vi "Advance past Number.vi"(7 "JSON":string, 9 "Offset (0)":i32, 11 "Parser State in":T2=enum."Number/Other") -> (1 "Offset past match":i32, 3 "Parser State":T2, 4 "JSON Value Type":T1, 6 "Value start out":i32)   [LabVIEW 2019, in "JSONtext.lvlib"]
uses:
  JSONtext.lvlib
  Parsing State.ctl
  JSON Value Type.ctl
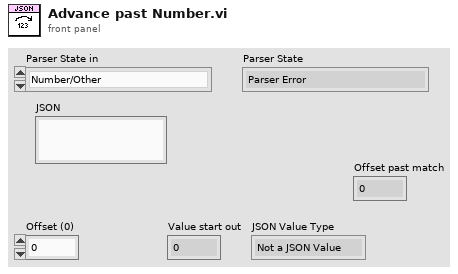
[diagram p1: front panel]
types:
  T1 = typedef "JSONtext.lvlib/JSON Value Type.ctl" = enum16{"Not a JSON Value", "JSON Object", "JSON Array", "String", "Number", "true", "false", "null"}
  T2 = typedef "JSONtext.lvlib/Parsing State.ctl" = enum16{"Parser Error", "Object", "Array", "String", "Number/Other", "Leading Whitespace", "Object end", "Array end", "Value end"}
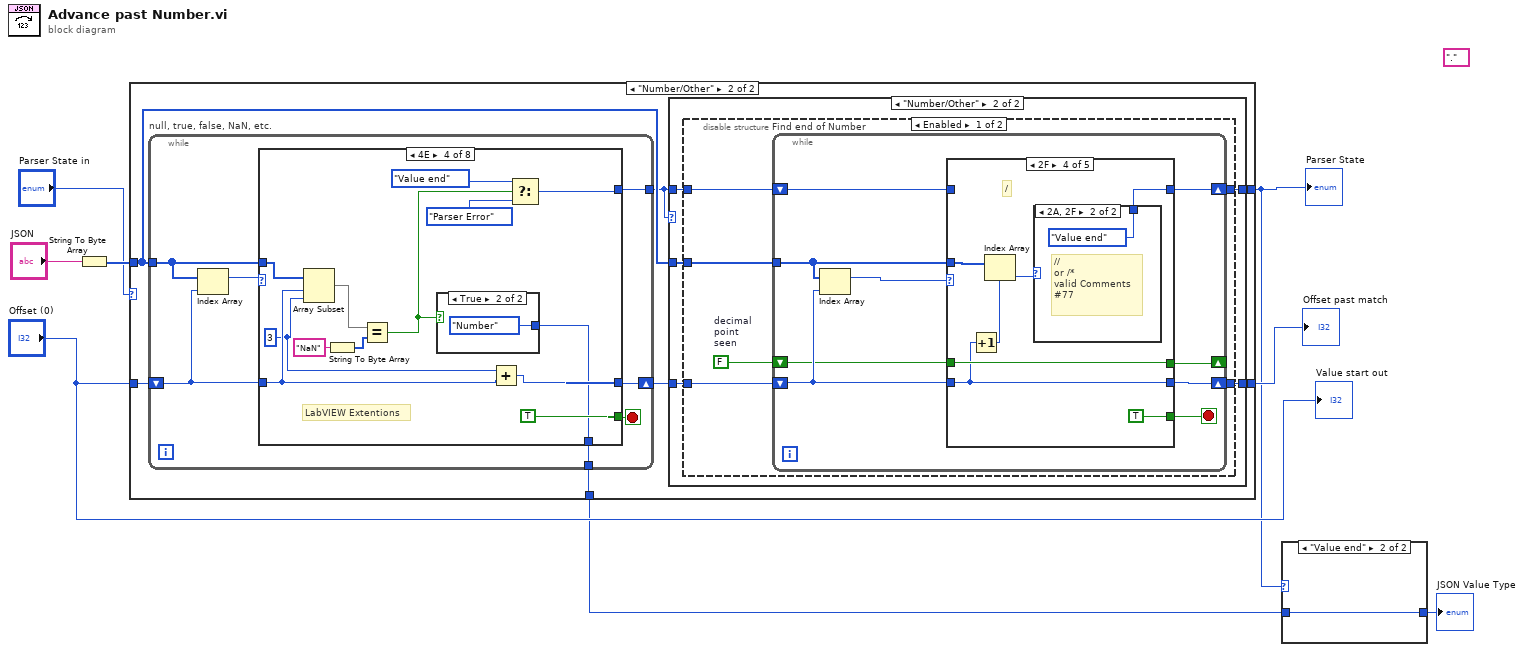
[diagram p0: block diagram]
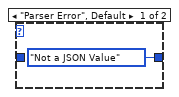
[diagram p2: hidden frame]
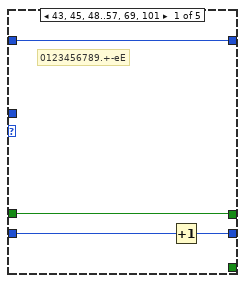
[diagram p5: hidden frame]
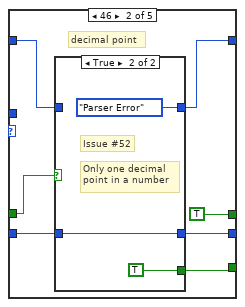
[diagram p6: hidden frame]
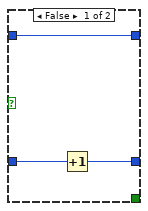
[diagram p7: hidden frame]
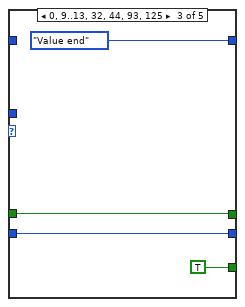
[diagram p8: hidden frame]
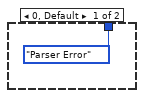
[diagram p9: hidden frame]
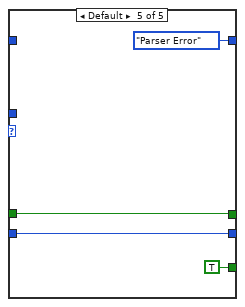
[diagram p10: hidden frame]
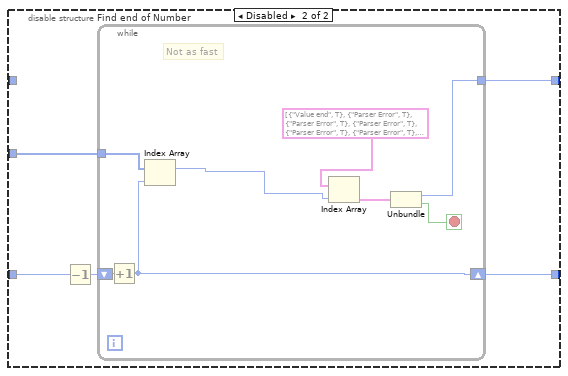
[diagram p11: hidden frame]
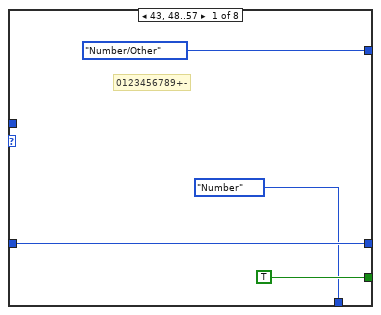
[diagram p12: hidden frame]
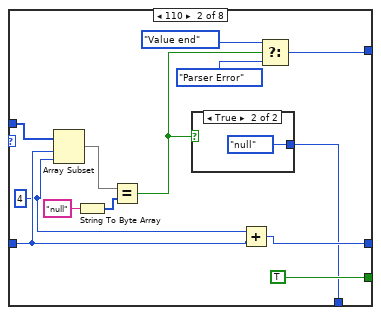
[diagram p13: hidden frame]
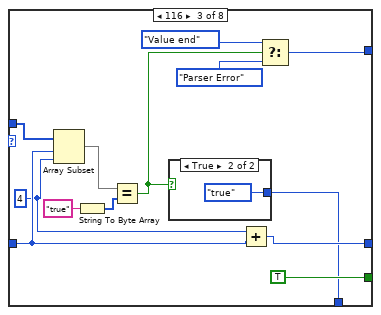
[diagram p15: hidden frame]
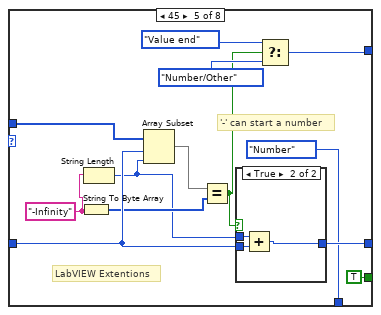
[diagram p18: hidden frame]
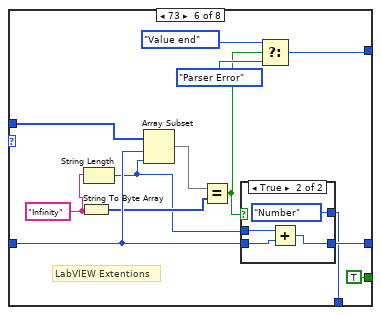
[diagram p20: hidden frame]
diagram:
  (unwired) "."
  n1 = String To Byte Array(string="JSON") -> (unsigned byte array=w5:u8[])
  n2 = case shown="\"Number/Other\"" "Parser State in" {
    tunnel: [_ w16] -> w3
    tunnel: [w9 w15] -> w8
    tunnel: w5 -> [_ w13]
    tunnel: "Offset (0)" -> [w9 w11]
    tunnel: [_ w10] -> w2
    frame "Parser Error", Default {
    }
    frame "Number/Other" {
      n3 = while "null, true, false, NaN, etc." {
        tunnel: w13 -> [w91]
        shift-right: [w87] -> w14
        shift-left: w11 -> [w88]
        tunnel: [w90] -> w12
        tunnel: [w86] -> w10
        stop <- w89 stop-if-true
        n4 = Index Array(array=w91, index=w88) -> (element=w92:u8)
        n5 = case shown="4E" w92 {
          tunnel: w91 -> [_ w108 w122 w136 w151 w168 w185 _]
          tunnel: [Parsing_State."Number/Other" w105 w119 w133 w149 w166 w182 Parsing_State."Parser Error"] -> w90
          tunnel: [TRUE TRUE TRUE TRUE TRUE TRUE TRUE TRUE] -> w89
          tunnel: w88 -> [w94 w101 w115 w129 w145 w162 w178 w191]
          tunnel: [w94 w99 w113 w127 w144 w161 w176 w191] -> w87
          tunnel: [JSON_Value_Type."Number" w97 w111 w125 JSON_Value_Type."Number" w156 w174 JSON_Value_Type."Not a JSON Value"] -> w86
          frame 43, 48..57 {
            # "0123456789+-"
          }
          frame 110 {
            w100 = 4 ("length")
            n6 = Array Subset(array=w108, index=w101, length=w100) -> (w106:u8[])
            n7 = String To Byte Array(string="null") -> (unsigned byte array=w107:u8[])
            n8 = Equal?(x=w106, y=w107) -> (x = y?=w98:bool)
            n9 = case shown="True" w98 {
              tunnel: [_ JSON_Value_Type."null"] -> w97
              frame False {
              }
              frame True {
              }
            }
            n10 = Add(x=w100, y=w101) -> (x+y=w99:i32)
            n11 = Select(t=Parsing_State."Value end", s=w98, f=Parsing_State."Parser Error") -> (s? t:f=w105:T2)
          }
          frame 116 {
            w114 = 4 ("length")
            n12 = Array Subset(array=w122, index=w115, length=w114) -> (w120:u8[])
            n13 = String To Byte Array(string="true") -> (unsigned byte array=w121:u8[])
            n14 = Equal?(x=w120, y=w121) -> (x = y?=w112:bool)
            n15 = case shown="True" w112 {
              tunnel: [_ JSON_Value_Type."true"] -> w111
              frame False {
              }
              frame True {
              }
            }
            n16 = Add(x=w114, y=w115) -> (x+y=w113:i32)
            n17 = Select(t=Parsing_State."Value end", s=w112, f=Parsing_State."Parser Error") -> (s? t:f=w119:T2)
          }
          frame 78 {
            w128 = 3 ("length")
            # "LabVIEW Extentions"
            n18 = Array Subset(array=w136, index=w129, length=w128) -> (w134:u8[])
            n19 = String To Byte Array(string="NaN") -> (unsigned byte array=w135:u8[])
            n20 = Equal?(x=w134, y=w135) -> (x = y?=w126:bool)
            n21 = case shown="True" w126 {
              tunnel: [_ JSON_Value_Type."Number"] -> w125
              frame False {
              }
              frame True {
              }
            }
            n22 = Add(x=w128, y=w129) -> (x+y=w127:i32)
            n23 = Select(t=Parsing_State."Value end", s=w126, f=Parsing_State."Parser Error") -> (s? t:f=w133:T2)
          }
          frame 45 {
            w142 = "-Infinity"
            # "'-' can start a number"
            # "LabVIEW Extentions"
            n24 = String To Byte Array(string=w142) -> (unsigned byte array=w143:u8[])
            n25 = String Length(string=w142) -> (length=w141:i32)
            n26 = Array Subset(array=w151, index=w145, length=w141) -> (w150:u8[])
            n27 = Equal?(x=w150, y=w143) -> (x = y?=w140:bool)
            n28 = case shown="True" w140 {
              tunnel: w145 -> [w152 w155]
              tunnel: [w152 w154] -> w144
              tunnel: w141 -> [_ w153]
              frame False {
              }
              frame True {
                n29 = Add(x=w153, y=w155) -> (x+y=w154:i32)
              }
            }
            n30 = Select(t=Parsing_State."Value end", s=w140, f=Parsing_State."Number/Other") -> (s? t:f=w149:T2)
          }
          frame 73 {
            w159 = "Infinity"
            # "LabVIEW Extentions"
            n31 = String To Byte Array(string=w159) -> (unsigned byte array=w160:u8[])
            n32 = String Length(string=w159) -> (length=w158:i32)
            n33 = Array Subset(array=w168, index=w162, length=w158) -> (w167:u8[])
            n34 = Equal?(x=w167, y=w160) -> (x = y?=w157:bool)
            n35 = case shown="True" w157 {
              tunnel: w162 -> [w169 w173]
              tunnel: [w169 w172] -> w161
              tunnel: w158 -> [_ w171]
              tunnel: [_ JSON_Value_Type."Number"] -> w156
              frame False {
              }
              frame True {
                n36 = Add(x=w171, y=w173) -> (x+y=w172:i32)
              }
            }
            n37 = Select(t=Parsing_State."Value end", s=w157, f=Parsing_State."Parser Error") -> (s? t:f=w166:T2)
          }
          frame 102 {
            w177 = 5 ("length")
            n38 = Array Subset(array=w185, index=w178, length=w177) -> (w183:u8[])
            n39 = String To Byte Array(string="false") -> (unsigned byte array=w184:u8[])
            n40 = Equal?(x=w183, y=w184) -> (x = y?=w175:bool)
            n41 = case shown="True" w175 {
              tunnel: [_ JSON_Value_Type."false"] -> w174
              frame False {
              }
              frame True {
              }
            }
            n42 = Add(x=w177, y=w178) -> (x+y=w176:i32)
            n43 = Select(t=Parsing_State."Value end", s=w175, f=Parsing_State."Parser Error") -> (s? t:f=w182:T2)
          }
          frame Default {
          }
        }
      }
      n44 = case shown="\"Number/Other\"" w12 {
        tunnel: [w17 w23] -> w16
        tunnel: [w18 w22] -> w15
        tunnel: w14 -> [w18 w19]
        tunnel: w12 -> [w17 w21]
        tunnel: w13 -> [_ w20]
        frame "Parser Error", Default {
        }
        frame "Number/Other" {
          n45 = disable-structure shown="Enabled" {
            disable-tunnel: [w29 w77] -> w23
            disable-tunnel: [w28 w76] -> w22
            disable-tunnel: w21 -> [w27 _]
            disable-tunnel: w20 -> [w26 w75]
            disable-tunnel: w19 -> [w25 w74]
            frame Enabled {
              w24 = FALSE  # decimal point seen
              n46 = while "Find end of Number" {
                tunnel: w26 -> [w38]
                shift-right: [w34] -> w28
                shift-left: w25 -> [w32]
                shift-right: [w36] -> w29
                shift-left: w27 -> [w37]
                shift-right: [w31] -> _
                shift-left: w24 -> [w30]
                stop <- w35 stop-if-true
                n47 = Index Array(array=w38, index=w32) -> (element=w33:u8)
                n48 = case shown="2F" w33 {
                  tunnel: w38 -> [_ _ _ w62 _]
                  tunnel: w37 -> [w42 w45 _ _ _]
                  tunnel: [w42 w44 Parsing_State."Value end" w60 Parsing_State."Parser Error"] -> w36
                  tunnel: [_ w43 TRUE TRUE TRUE] -> w35
                  tunnel: w32 -> [w41 w49 w57 w64 w72]
                  tunnel: [w40 w48 w57 w64 w72] -> w34
                  tunnel: [w39 TRUE w56 w65 w69] -> w31
                  tunnel: w30 -> [w39 w46 w56 w65 w69]
                  frame 43, 45, 48..57, 69, 101 {
                    # "0123456789.+-eE"
                    n49 = Increment(x=w41) -> (x+1=w40:i32)
                  }
                  frame 46 {
                    # "decimal point"
                    n50 = case shown="True" w46 {
                      tunnel: w49 -> [w52 w54]
                      tunnel: [w51 w54] -> w48
                      tunnel: [w50 Parsing_State."Parser Error"] -> w44
                      tunnel: w45 -> [w50 _]
                      tunnel: [_ TRUE] -> w43
                      frame False {
                        n51 = Increment(x=w52) -> (x+1=w51:i32)
                      }
                      frame True {
                        # "Only one decimal\npoint in a number"
                        # "Issue #52"
                      }
                    }
                  }
                  frame 0, 9..13, 32, 44, 93, 125 {
                  }
                  frame 47 {
                    # "/"
                    n52 = Increment(x=w64) -> (x+1=w63:i32)
                    n53 = Index Array(array=w62, index=w63) -> (element=w61:u8)
                    n54 = case shown="2A, 2F" w61 {
                      tunnel: [Parsing_State."Parser Error" Parsing_State."Value end"] -> w60
                      frame 0, Default {
                      }
                      frame 42, 47 {
                        # "//\nor /*\nvalid Comments\n#77"
                      }
                    }
                  }
                  frame Default {
                  }
                }
              }
            }
            frame Disabled {
              n55 = Decrement(x=w74) -> (x-1=w73:i32)
              n56 = while "Find end of Number" {
                tunnel: w75 -> [w85]
                shift-right: [w78] -> w76
                shift-left: w73 -> [w84]
                tunnel: [w79] -> w77
                stop <- w80 stop-if-true
                # "Not as fast"
                n57 = Increment(x=w84) -> (x+1=w78:i32)
                n58 = Index Array(array=w85, index=w78) -> (element=w81:u8)
                n59 = Index Array(array=cluster{T2, bool}[] [{enum."Value end", TRUE}, {enum."Parser Error", TRUE}, {enum."Parser Error", TRUE}, {enum."Parser Error", TRUE}, {enum."Parser Error", TRUE}, {enum."Parser Error", TRUE}, {enum."Parser Error", TRUE}, {enum."Parser Error", TRUE}, {enum."Parser Error", TRUE}, {enum."Value end", TRUE}, {enum."Value end", TRUE}, {enum."Value end", TRUE}, {enum."Value end", TRUE}, {enum."Value end", TRUE}, {enum."Parser Error", TRUE}, {enum."Parser Error", TRUE}, {enum."Parser Error", TRUE}, {enum."Parser Error", TRUE}, {enum."Parser Error", TRUE}, {enum."Parser Error", TRUE}, {enum."Parser Error", TRUE}, {enum."Parser Error", TRUE}, {enum."Parser Error", TRUE}, {enum."Parser Error", TRUE}, {enum."Parser Error", TRUE}, {enum."Parser Error", TRUE}, {enum."Parser Error", TRUE}, {enum."Parser Error", TRUE}, {enum."Parser Error", TRUE}, {enum."Parser Error", TRUE}, {enum."Parser Error", TRUE}, {enum."Parser Error", TRUE}, {enum."Value end", TRUE}, {enum."Parser Error", TRUE}, {enum."Parser Error", TRUE}, {enum."Parser Error", TRUE}, {enum."Parser Error", TRUE}, {enum."Parser Error", TRUE}, {enum."Parser Error", TRUE}, {enum."Parser Error", TRUE}, {enum."Parser Error", TRUE}, {enum."Parser Error", TRUE}, {enum."Parser Error", TRUE}, {enum."Number/Other", FALSE}, {enum."Value end", TRUE}, {enum."Number/Other", FALSE}, {enum."Number/Other", FALSE}, {enum."Parser Error", TRUE}, {enum."Number/Other", FALSE}, {enum."Number/Other", FALSE}, {enum."Number/Other", FALSE}, {enum."Number/Other", FALSE}, {enum."Number/Other", FALSE}, {enum."Number/Other", FALSE}, {enum."Number/Other", FALSE}, {enum."Number/Other", FALSE}, {enum."Number/Other", FALSE}, {enum."Number/Other", FALSE}, {enum."Parser Error", TRUE}, {enum."Parser Error", TRUE}, {enum."Parser Error", TRUE}, {enum."Parser Error", TRUE}, {enum."Parser Error", TRUE}, {enum."Parser Error", TRUE}, {enum."Parser Error", TRUE}, {enum."Parser Error", TRUE}, {enum."Parser Error", TRUE}, {enum."Parser Error", TRUE}, {enum."Parser Error", TRUE}, {enum."Number/Other", FALSE}, {enum."Parser Error", TRUE}, {enum."Parser Error", TRUE}, {enum."Parser Error", TRUE}, {enum."Parser Error", TRUE}, {enum."Parser Error", TRUE}, {enum."Parser Error", TRUE}, {enum."Parser Error", TRUE}, {enum."Parser Error", TRUE}, {enum."Parser Error", TRUE}, {enum."Parser Error", TRUE}, {enum."Parser Error", TRUE}, {enum."Parser Error", TRUE}, {enum."Parser Error", TRUE}, {enum."Parser Error", TRUE}, {enum."Parser Error", TRUE}, {enum."Parser Error", TRUE}, {enum."Parser Error", TRUE}, {enum."Parser Error", TRUE}, {enum."Parser Error", TRUE}, {enum."Parser Error", TRUE}, {enum."Parser Error", TRUE}, {enum."Parser Error", TRUE}, {enum."Parser Error", TRUE}, {enum."Value end", TRUE}, {enum."Parser Error", TRUE}, {enum."Parser Error", TRUE}, {enum."Parser Error", TRUE}, {enum."Parser Error", TRUE}, {enum."Parser Error", TRUE}, {enum."Parser Error", TRUE}, {enum."Parser Error", TRUE}, {enum."Number/Other", FALSE}, {enum."Parser Error", TRUE}, {enum."Parser Error", TRUE}, {enum."Parser Error", TRUE}, {enum."Parser Error", TRUE}, {enum."Parser Error", TRUE}, {enum."Parser Error", TRUE}, {enum."Parser Error", TRUE}, {enum."Parser Error", TRUE}, {enum."Parser Error", TRUE}, {enum."Parser Error", TRUE}, {enum."Parser Error", TRUE}, {enum."Parser Error", TRUE}, {enum."Parser Error", TRUE}, {enum."Parser Error", TRUE}, {enum."Parser Error", TRUE}, {enum."Parser Error", TRUE}, {enum."Parser Error", TRUE}, {enum."Parser Error", TRUE}, {enum."Parser Error", TRUE}, {enum."Parser Error", TRUE}, {enum."Parser Error", TRUE}, {enum."Parser Error", TRUE}, {enum."Parser Error", TRUE}, {enum."Value end", TRUE}] ("Array"), index=w81) -> (element=w82:cluster{T2, bool})
                n60 = Unbundle(w82) -> (w79:T2, w80:bool)
              }
            }
          }
        }
      }
    }
  }
  "Parser State" <- w3
  "Offset past match" <- w8
  n61 = case shown="\"Value end\"" w3 {
    tunnel: w2 -> [_ w193]
    tunnel: [JSON_Value_Type."Not a JSON Value" w193] -> w1
    frame "Parser Error", Default {
    }
    frame "Value end" {
    }
  }
  "JSON Value Type" <- w1
  "Value start out" <- "Offset (0)"
